vi "Rinocloud_ancestors_JSON_parsing.vi"(3 "error in (no error)":errorcluster, 5 "JSON string":string) -> (0 "error out":errorcluster, 1 "last ID":string, 2 "metadata array":T1(array[cluster]))   [LabVIEW 2011, in "Rinocloud Library.lvlib"]
uses:
  Rinocloud Library.lvlib
  i3 JSON/i3-json.lvlib
  i3 JSON/JSON Parsing/Get Object Parameter Files/Get Object Parameter - Numeric.vi
  i3 JSON/JSON Parsing/Get Object Parameter Files/Get Object Parameter - String.vi
  i3 JSON/JSON Parsing/Get Object Parameter Files/Get Object Parameter - Array.vi
  i3 JSON/JSON Parsing/Get Array Value at Index Files/Get Array Value at Index - Array.vi
  i3 JSON/JSON Parsing/Get Array Value at Index Files/Get Array Value at Index - String.vi
  i3 JSON/JSON Parsing/Get Object Parameter Files/Get Object Parameter - Object.vi
panel:
  out "JSON Tree Passthrough (JSON Array)":variant
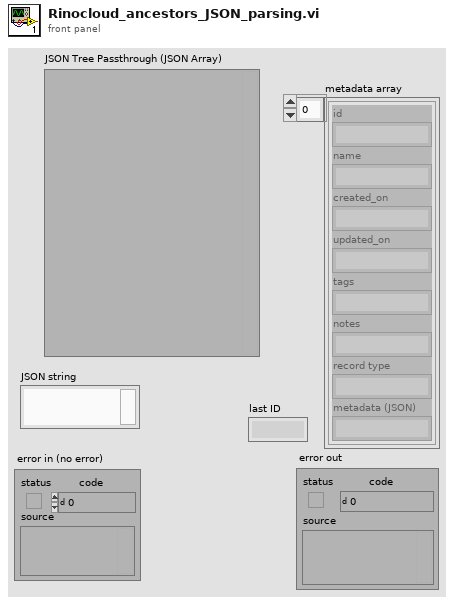
[diagram p1: front panel]
types:
  T1 = cluster{"id":string, "name":string, "created_on":string, "updated_on":string, "tags":string, "notes":string, "record type":string, "metadata (JSON)":string}[]
  T2 = cluster{"id":string, "name":string, "created_on":string, "updated_on":string, "tags":string, "notes":string, "record type":string, "metadata (JSON)":string}
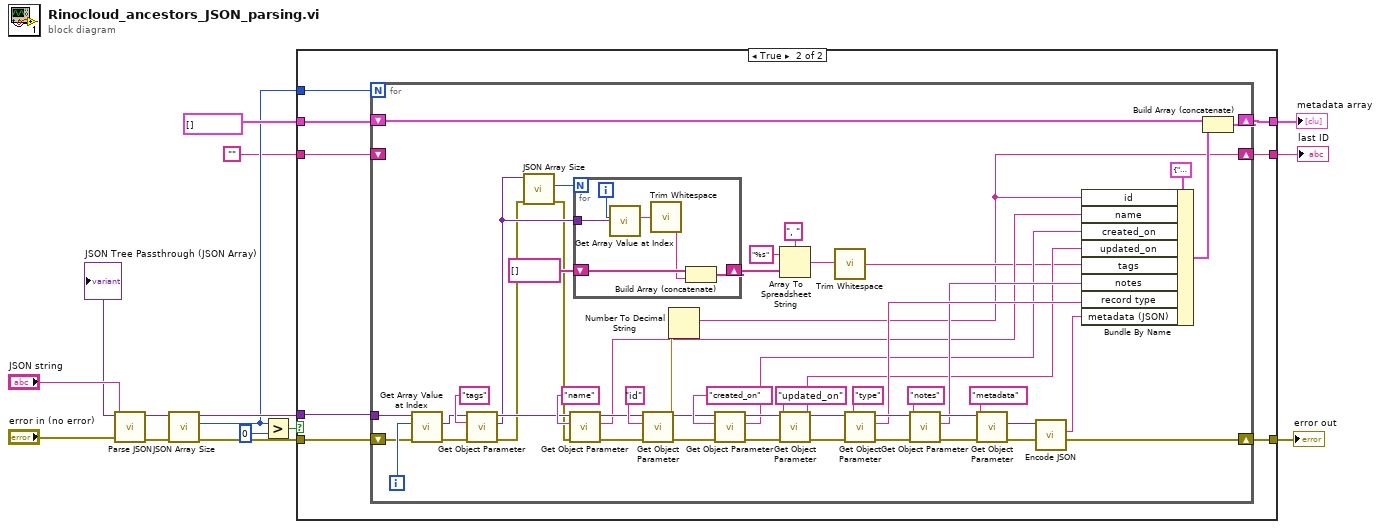
[diagram p0: block diagram]
diagram:
  n1 = call "Parse JSON.vi"("error in (no error)"="error in (no error)", "JSON String"="JSON string") -> ("error out"=w8:errorcluster, "JSON Tree"=w7:variant)  [unwired: 6 in, 2 out]
  n2 = call "JSON Array Size.vi"("error in (no error)"=w8, "JSON Tree In (JSON Array)"=w7) -> ("error out"=w5:errorcluster, "Array Size"=w4:i32, "JSON Tree Passthrough (JSON Array)"=w6:variant)  [unwired: 7 in]
  "JSON Tree Passthrough (JSON Array)" <- w6
  n3 = Greater?(x=w4, y=0) -> (0:w11:bool)
  n4 = case shown="True" w11 {
    tunnel: w5 -> [w16 w20]
    tunnel: w6 -> [_ w21]
    tunnel: w4 -> [_ w25]
    tunnel: [w16 w24] -> w13
    tunnel: [w17 w23] -> w10
    tunnel: T1 [] -> [w17 w22]
    tunnel: "" -> [w15 w19]
    tunnel: [w15 w18] -> w1
    frame False {
    }
    frame True {
      n5 = for {
        N: w25 -> [_]
        tunnel: w21 -> [w74]
        shift-right: [w54] -> w24
        shift-left: w20 -> [w68]
        shift-right: [w33] -> w23
        shift-left: w22 -> [w31]
        shift-right: [w26] -> w18
        shift-left: w19 -> [_]
        i -> [w75]
        n6 = call-poly "Get Array Value at Index.vi"("error in (no error)"=w68, "Index"=w75, "JSON Tree In (JSON Array)"=w74) -> ("error out"=w44:errorcluster, "JSON Array"=w29:variant)  [unwired: 5 in, 2 out]
        n7 = call-poly "Get Object Parameter.vi"("error in (no error)"=w44, "Parameter Name"="tags", "JSON Tree In (JSON Object)"=w29) -> ("error out"=w42:errorcluster, "JSON Array"=w43:variant, "JSON Tree Out Passthrough"=w45:variant)  [unwired: 5 in, 1 out]
        n8 = call "JSON Array Size.vi"("error in (no error)"=w42, "JSON Tree In (JSON Array)"=w43) -> ("error out"=w41:errorcluster, "Array Size"=w51:i32)  [unwired: 7 in, 1 out]
        n9 = call-poly "Get Object Parameter.vi"("error in (no error)"=w41, "Parameter Name"="name", "JSON Tree In (JSON Object)"=w45) -> ("error out"=w67:errorcluster, "String Value"=w30:string, "JSON Tree Out Passthrough"=w72:variant)  [unwired: 5 in, 1 out]
        n10 = for {
          N: w51 -> [_]
          tunnel: w43 -> [w82]
          shift-right: [w80] -> w47
          shift-left: string[] [] ("Tags 2") -> [w81]
          i -> [w79]
          n11 = call-poly "Get Array Value at Index.vi"("Index"=w79, "JSON Tree In (JSON Array)"=w82) -> ("String Value"=w78:string)  [unwired: 6 in, 3 out]
          n12 = call <vilib>:"Trim Whitespace.vi"("string"=w78) -> ("trimmed string"=w77:string)  [unwired: 1 in]
          n13 = Build Array (concatenate)(w81, w77) -> (w80:string[])
        }
        n14 = call-poly "Get Object Parameter.vi"("error in (no error)"=w67, "Parameter Name"="id", "JSON Tree In (JSON Object)"=w72) -> ("error out"=w57:errorcluster, "Double Value"=w53:dbl, "JSON Tree Out Passthrough"=w58:variant)  [unwired: 5 in, 1 out]
        n15 = Number To Decimal String(number=w53) -> (decimal integer string=w26:string)  [unwired: 1 in]
        n16 = call-poly "Get Object Parameter.vi"("error in (no error)"=w57, "Parameter Name"="created_on", "JSON Tree In (JSON Object)"=w58) -> ("error out"=w55:errorcluster, "String Value"=w34:string, "JSON Tree Out Passthrough"=w56:variant)  [unwired: 5 in, 1 out]
        n17 = Array To Spreadsheet String(delimiter (Tab)=", ", array=w47, 3:"%s" ("format string")) -> (spreadsheet string=w28:string)
        n18 = call-poly "Get Object Parameter.vi"("error in (no error)"=w55, "Parameter Name"="updated_on", "JSON Tree In (JSON Object)"=w56) -> ("error out"=w66:errorcluster, "String Value"=w35:string, "JSON Tree Out Passthrough"=w69:variant)  [unwired: 5 in, 1 out]
        n19 = call <vilib>:"Trim Whitespace.vi"("string"=w28) -> ("trimmed string"=w27:string)  [unwired: 1 in]
        n20 = call-poly "Get Object Parameter.vi"("error in (no error)"=w66, "Parameter Name"="type", "JSON Tree In (JSON Object)"=w69) -> ("error out"=w39:errorcluster, "String Value"=w37:string, "JSON Tree Out Passthrough"=w40:variant)  [unwired: 5 in, 1 out]
        n21 = call-poly "Get Object Parameter.vi"("error in (no error)"=w39, "Parameter Name"="notes", "JSON Tree In (JSON Object)"=w40) -> ("error out"=w61:errorcluster, "String Value"=w36:string, "JSON Tree Out Passthrough"=w64:variant)  [unwired: 5 in, 1 out]
        n22 = call-poly "Get Object Parameter.vi"("error in (no error)"=w61, "Parameter Name"="metadata", "JSON Tree In (JSON Object)"=w64) -> ("error out"=w60:errorcluster, "JSON Object"=w62:variant)  [unwired: 5 in, 2 out]
        n23 = call "Encode JSON.vi"("error in (no error)"=w60, "JSON Tree"=w62) -> ("error out"=w54:errorcluster, "String"=w38:string)  [unwired: 4 in]
        n24 = Bundle By Name(cluster=T2 {"id"="", "name"="", "created_on"="", "updated_on"="", "tags"="", "notes"="", "record type"="", "metadata (JSON)"=""} ("metadata 2"), "id"=w26, "name"=w30, "created_on"=w34, "updated_on"=w35, "tags"=w27, "notes"=w36, "record type"=w37, "metadata (JSON)"=w38) -> (w32:T2)
        n25 = Build Array (concatenate)(w31, w32) -> (w33:T1)
      }
    }
  }
  "error out" <- w13
  "metadata array" <- w10
  "last ID" <- w1
